vi "GraphsUpdateMeanCam.vi"(9 "Old mean data in":dbl[][](array[numeric]), 10 "run data in":i32[][](array[numeric]), 11 "GraphChart in":refnum<vi>) -> (1 "New mean data out":dbl[][](array[numeric]))   [LabVIEW 2019]
uses:
  <vilib>/Analysis/baseanly.llb/Mean (DBL).vi
  controls/GlobalExp.vi
  <vilib>/Analysis/NI_AALBase.lvlib
  Global.lvlib
panel:
  out "Waveform Graph":dbl[][](graph)
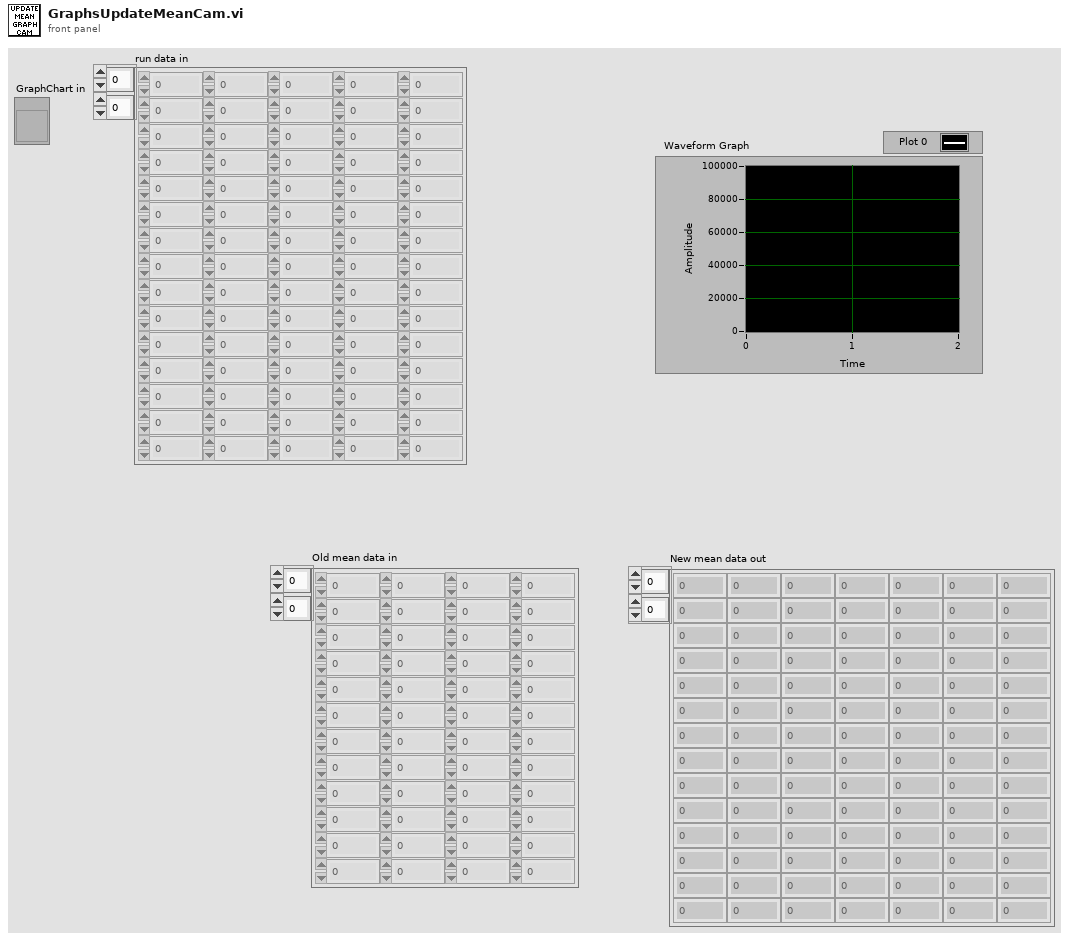
[diagram p1: front panel]
types:
  T1 = typedef "MasterExpControl.ctl" = cluster{"Main Steps":dbl, "Main Runs":dbl, "ExpStatus":enum16{"Innit", "Stop", "Idle", "MainRunning", "AuxRunning"}, "Main Current Step":dbl, "ExpNum":dbl, "NewData":bool, "date":string, "command":string, "Stop":bool, "Pause":bool, "Mathematica":string, "Main/Meta":bool, "UpdateMath":bool, "Camera":bool, "MetaExpOver":bool, "NextMetaExp":bool}
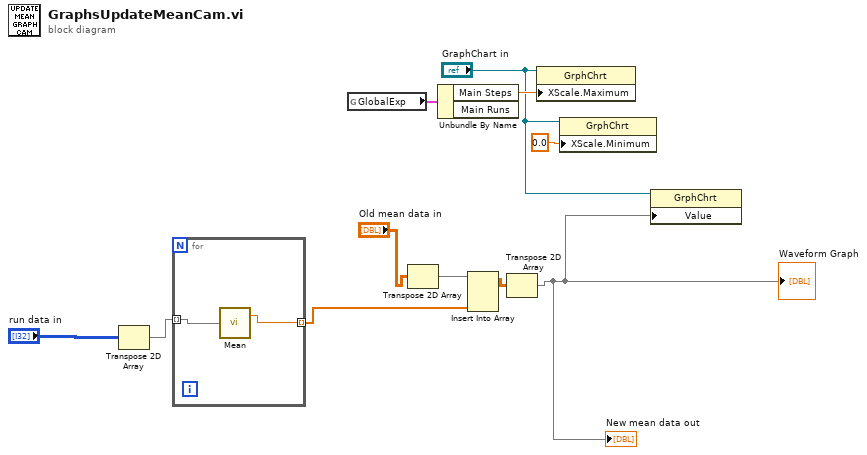
[diagram p0: block diagram]
diagram:
  n1 = Transpose 2D Array(2D array="run data in") -> (transposed array=w7:i32[][])
  n2 = for {
    tunnel: w7 -> [w13] mode=indexing
    tunnel: [w12] -> w6 mode=indexing
    n3 = call-poly <vilib>:"Mean.vi"("X"=w13) -> ("mean"=w12:dbl)  [unwired: 1 out]
  }
  n4 = global read "GlobalExp.vi" "GlobalExp"() -> (w11:T1)
  n5 = Transpose 2D Array(2D array="Old mean data in") -> (transposed array=w1:dbl[][])
  n6 = Unbundle By Name(w11) -> ("Main Steps"=w10:dbl)  [unwired: 1 out]
  n7 = Insert Into Array(array=w1, new element=w6) -> (w4:dbl[][])  [unwired: 2 in]
  n8 = Transpose 2D Array(2D array=w4) -> (transposed array=w3:dbl[][])
  "Waveform Graph" <- w3
  "New mean data out" <- w3
  n9 = property class="GrphChrt"(reference="GraphChart in", "XScale.Maximum"=w10) -> ()  [unwired: 1 in, 2 out]
  n10 = property class="GrphChrt"(reference="GraphChart in", "XScale.Minimum"=0.0 ("X Scale.Range:Minimum")) -> ()  [unwired: 1 in, 2 out]
  n11 = property class="GrphChrt"(reference="GraphChart in", "Value"=w3) -> ()  [unwired: 1 in, 2 out]
